vi "log jl exceptions.vi"(5 "log exception":bool, 7 "jl error info":T1) -> (3 "dup jl error info":T1)   [LabVIEW 2018, in "LV2Julia_core.lvlib"]
uses:
  LV2Julia_core.lvlib
  detailed error info.ctl
  StackFrame.ctl
  timestamped jl err info.ctl
  jl stack traces global.vi
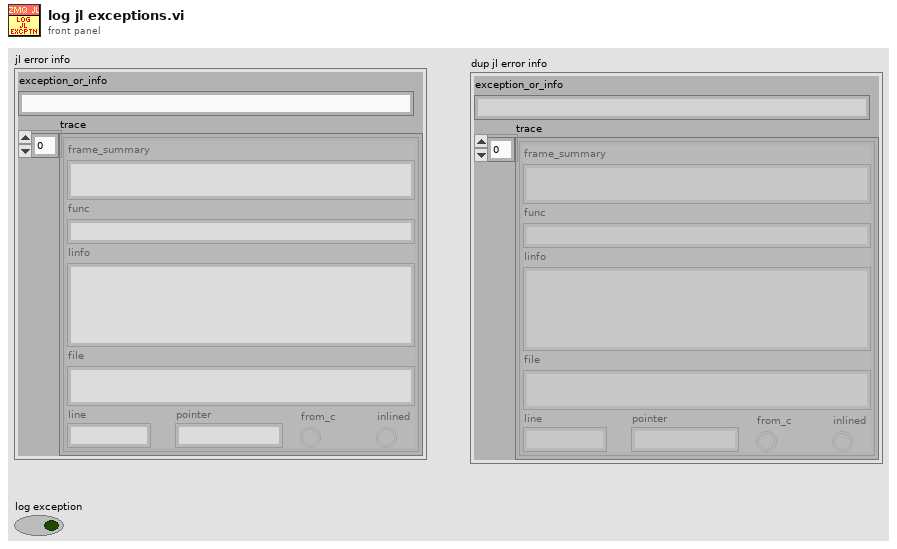
[diagram p1: front panel]
types:
  T1 = typedef "LV2Julia_core.lvlib/detailed error info.ctl" = cluster{"exception_or_info":string, "trace":T2[]}
  T2 = typedef "LV2Julia_core.lvlib/StackFrame.ctl" = cluster{"frame_summary":string, "func":string, "linfo":string, "file":string, "line":i32, "pointer":u64, "from_c":bool, "inlined":bool}
  T3 = typedef "LV2Julia_core.lvlib/timestamped jl err info.ctl" = cluster{"Time Stamp":timestamp, "detailed error info":T1}
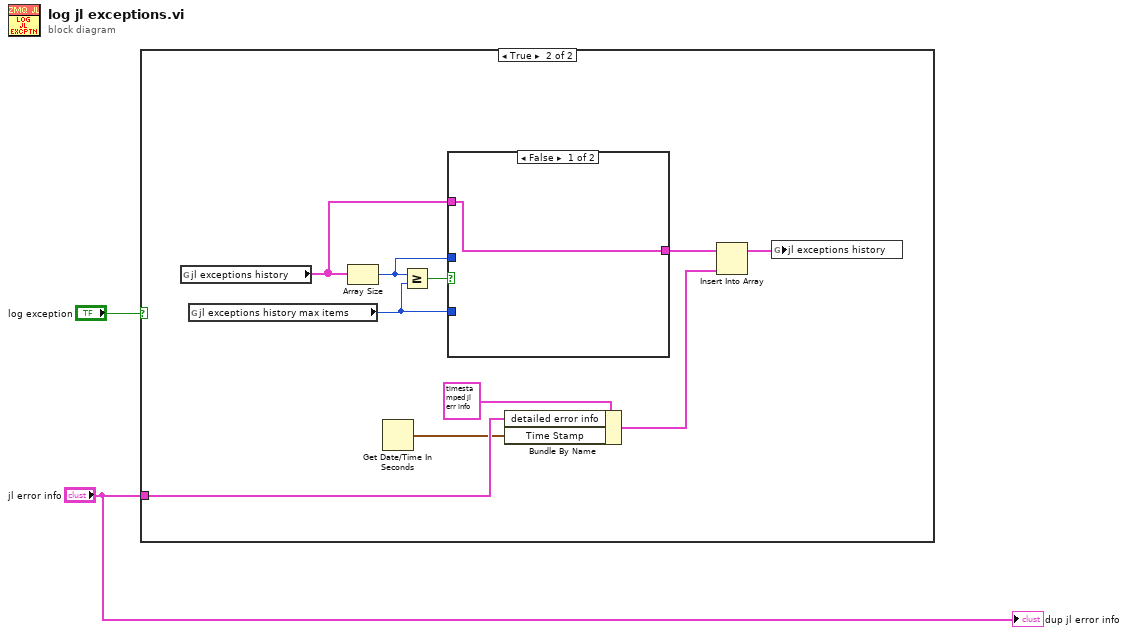
[diagram p0: block diagram]
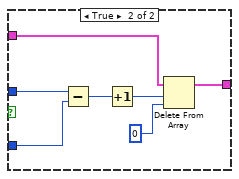
[diagram p3: hidden frame]
diagram:
  n1 = case shown="True" "log exception" {
    tunnel: "jl error info" -> [_ w5]
    frame False {
    }
    frame True {
      n2 = global read "jl stack traces global.vi" "jl exceptions history"() -> (w9:T3[])
      n3 = global read "jl stack traces global.vi" "jl exceptions history max items"() -> (w11:u32)
      n4 = Array Size(array=w9) -> (size(s)=w12:i32)
      n5 = Get Date/Time In Seconds() -> (seconds since 1Jan1904=w3:timestamp)
      n6 = Greater Or Equal?(x=w12, y=w11) -> (x >= y?=w10:bool)
      n7 = case shown="False" w10 {
        tunnel: w12 -> [_ w20]
        tunnel: w11 -> [_ w19]
        tunnel: w9 -> [w13 w17]
        tunnel: [w13 w14] -> w8
        frame False {
        }
        frame True {
          n8 = Subtract(x=w20, y=w19) -> (x-y=w18:u32)
          n9 = Increment(x=w18) -> (x+1=w15:u32)
          n10 = Delete From Array(array=w17, length=w15, index=0) -> (array with subset deleted=w14:T3[])  [unwired: 1 out]
        }
      }
      n11 = Bundle By Name(cluster=T3 {"Time Stamp"=timestamp(0 s since 1904-01-01), "detailed error info"={"exception_or_info"="", "trace"=[]}} ("timestamped jl err info"), "detailed error info"=w5, "Time Stamp"=w3) -> (w4:T3)
      n12 = Insert Into Array(array=w8, new element=w4) -> (w7:T3[])  [unwired: 1 in]
      n13 = global write "jl stack traces global.vi" "jl exceptions history"(w7) -> ()
    }
  }
  "dup jl error info" <- "jl error info"
